vi "5.3.vi"() -> ()   [LabVIEW 2017]
panel:
  out "数组":dbl[](array[numeric])
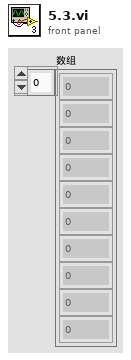
[diagram p1: front panel]
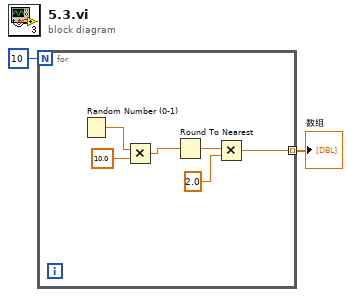
[diagram p0: block diagram]
diagram:
  n1 = for {
    N: 10 -> [_]
    tunnel: [w3] -> w1 mode=indexing
    n2 = Random Number (0-1)() -> (number: 0 to 1=w8:dbl)
    n3 = Multiply(x=w8, y=10.0) -> (x*y=w6:dbl)
    n4 = Round To Nearest(number=w6) -> (nearest integer value=w5:dbl)
    n5 = Multiply(x=w5, y=2.0) -> (x*y=w3:dbl)
  }
  "数组" <- w1
